vi "Global - System.vi"() -> ()   [LabVIEW 2019]
panel:
  out "System":T1(array[cluster])
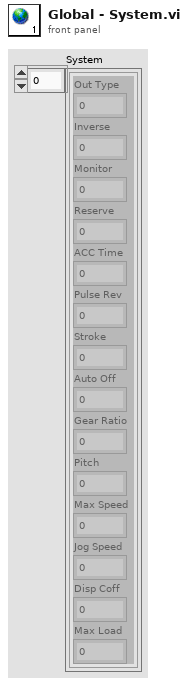
[diagram p1: front panel]
types:
  T1 = cluster{"Out Type":u8, "Inverse":u8, "Monitor":u8, "Reserve":u8, "ACC Time":u32, "Pulse Rev":u32, "Stroke":u32, "Auto Off":u32, "Gear Ratio":sgl, "Pitch":sgl, "Max Speed":u32, "Jog Speed":u32, "Disp Coff":sgl, "Max Load":u32}[]
diagram:
